vi "Init.vi"(5 "PathControl.lvclass":refnum<class "PathControl.lvclass">, 6 "Environmental classes":refnum<class "Instrument.lvclass">[](array[class]), 7 "XML Handler.lvclass":refnum<class "XML Handler.lvclass">, 8 "error in (no error)":errorcluster, 9 "Instruments to Use":T2(array[cluster]), 10 "Device.lvclass":refnum<class "Device.lvclass">, 11 "Measurements in":refnum<class "Measurement.lvclass">) -> (0 "error out":errorcluster, 3 "Measurements out":refnum<class "Measurement.lvclass">)   [LabVIEW 2020, in "Measurement.lvclass"]
doc: "Initializes the measurement.\nThis verifies that the instruments are present and adds them into the class data.\nIs also adds the xml handler into the class data."
uses:
  Measurement.lvclass
  Devices/Device.lvclass
  Instruments/Instrument.lvclass
  XML Handler/XML Handler.lvclass
  Path Control/PathControl.lvclass
  Path Control/Measurements Specific Paths.ctl
  Controls/Init States.ctl
  Instruments/Power Supply/Power Supply.lvclass
  Instruments/Temperature Control/Temperature Control.lvclass
  Instruments/Digital Multimeter/Digital Multimeter.lvclass
  Measurement.lvclass/Measurement.ctl
  Devices/Controls/Change setting mode enum.ctl
  Devices/PIC-device/PIC-Device.lvclass
panel:
  in  "Measurement specific paths":T1=enum."IMD"
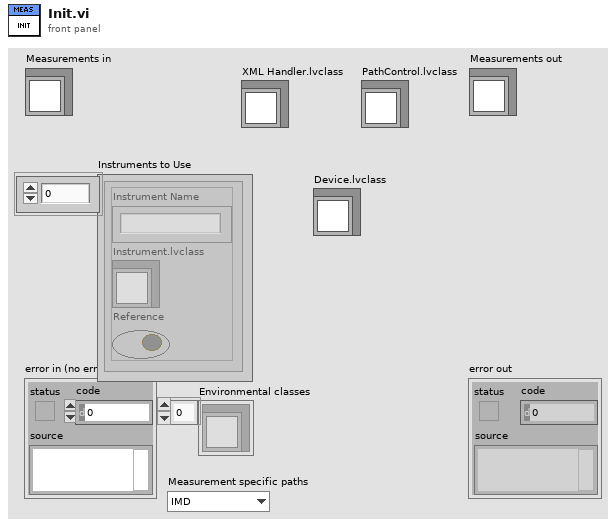
[diagram p1: front panel]
types:
  T1 = typedef "PathControl.lvclass/Measurements Specific Paths.ctl" = enum16{"No calibration", "Harmonics", "IMD", "S Parameter", "AM-AM", "MCCW-ACLR", "DC", "LCR", "Power Meter GUI", "RF Power"}
  T2 = cluster{"Instrument Name":string, "Instrument.lvclass":refnum<class "Instrument.lvclass">, "Reference":bool}[]
  T3 = typedef "Measurement.lvclass/Init States.ctl" = enum16{"Verify instruments", "Init Parameters", "Init Instruments", "Add Device", "Init Device", "Create test in XML", "Set path", "Done"}
  T4 = typedef "PIC-Device.lvclass/Change setting mode enum.ctl" = enum16{"Init", "Next", "Reset"}
  T5 = typedef "Device.lvclass/DC Offset Cluster.ctl" = cluster{"Enable":bool, "Use Array":bool, "Array":dbl[], "To From Cluster":cluster{"From":dbl, "To":dbl, "Step":dbl}, "Current Value":dbl, "DC Offset":refnum<class "Power Supply.lvclass">}
  T6 = typedef "Device.lvclass/Device Information Cluster.ctl" = cluster{"Device Info":string[][], "Default Values":T7[], "Fetched info":string[][]}
  T7 = typedef "PIC-Device.lvclass/Register to Write.ctl" = cluster{"Register":u32, "Value":u32, "Dev Address":u32, "Physical Adress":u32}
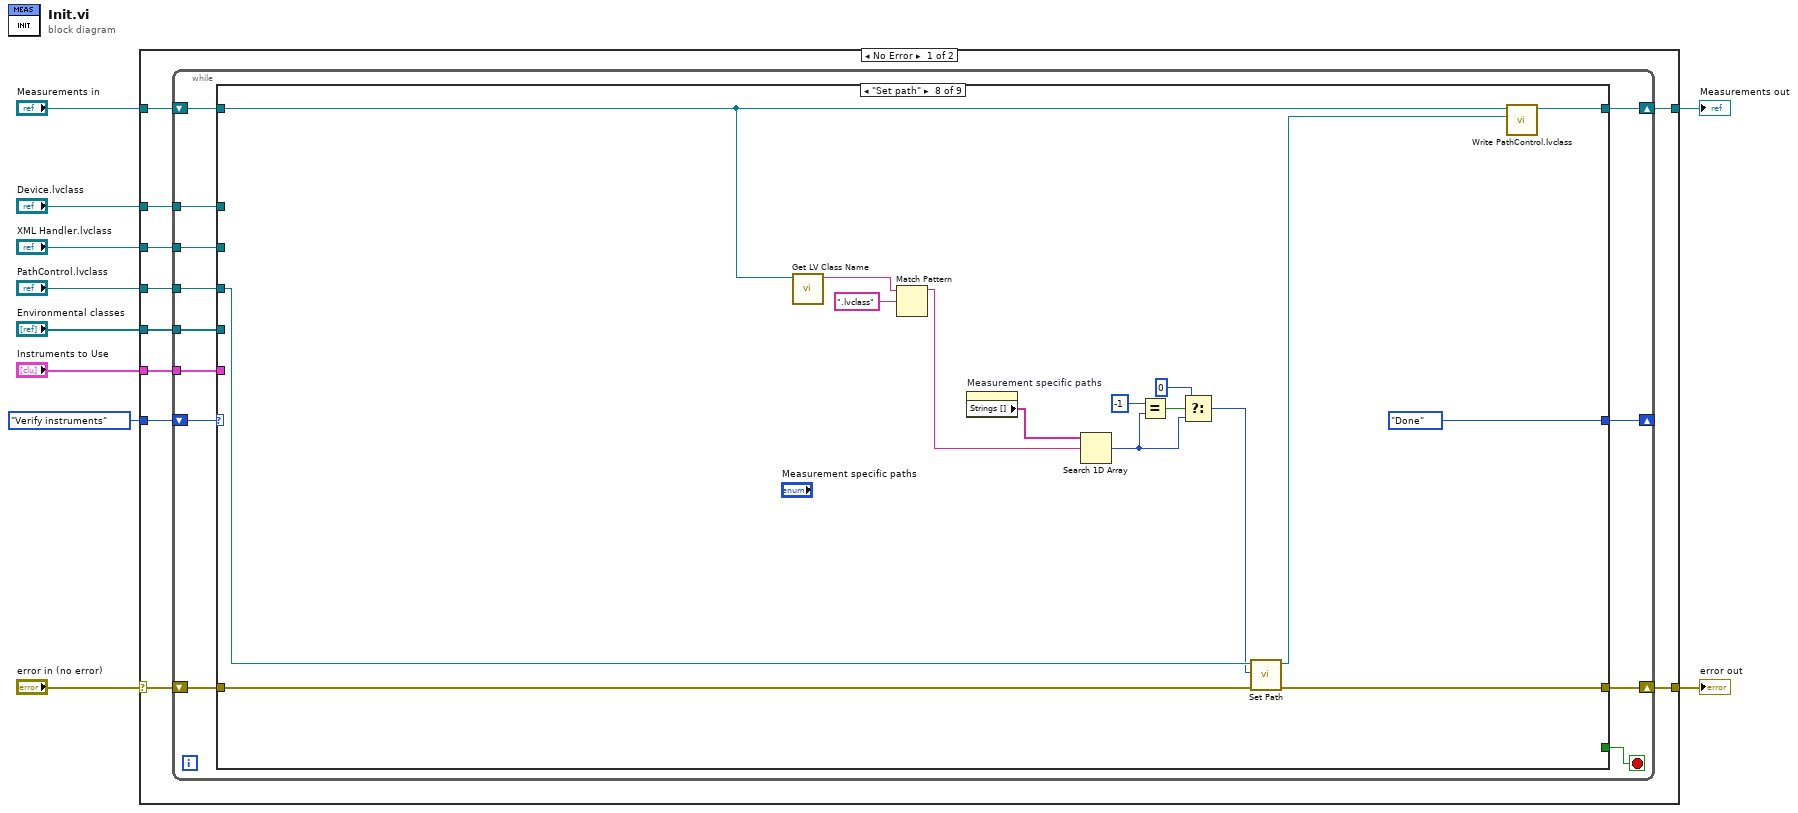
[diagram p0: block diagram]
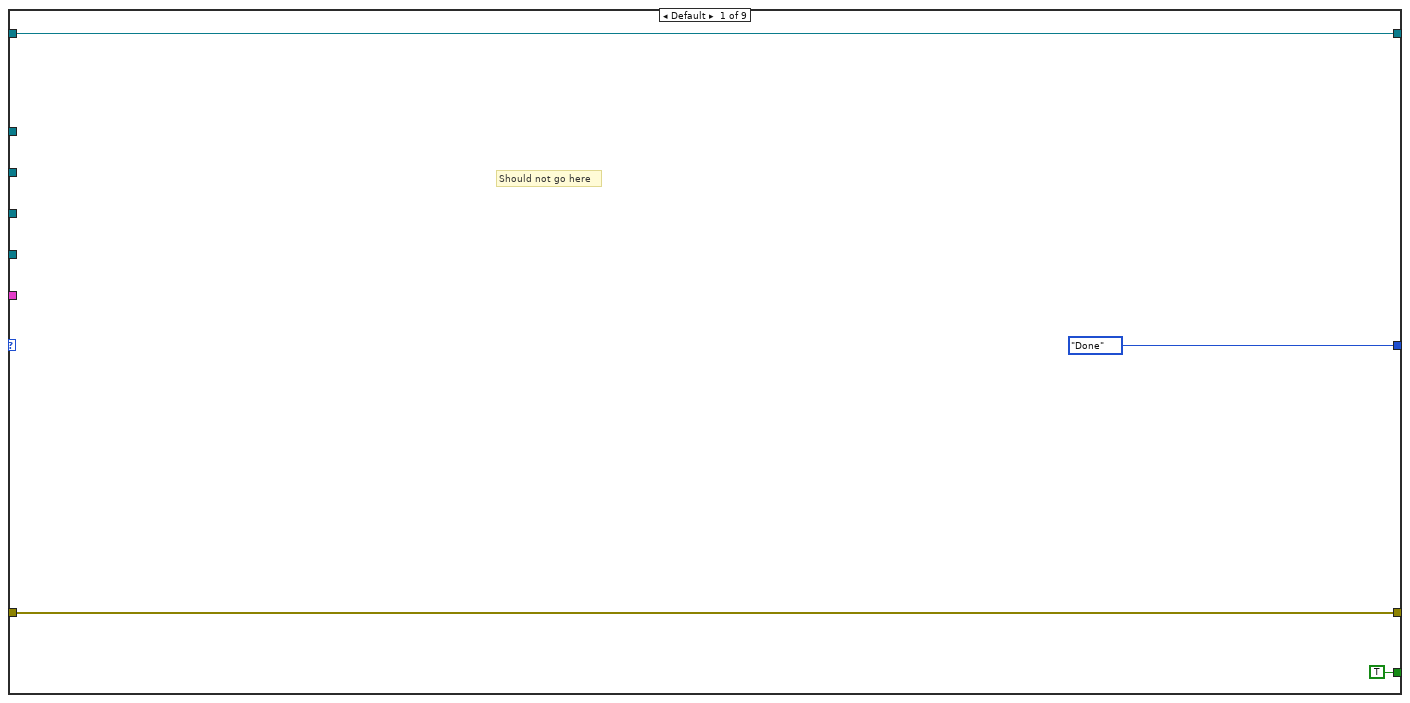
[diagram p2: hidden frame]
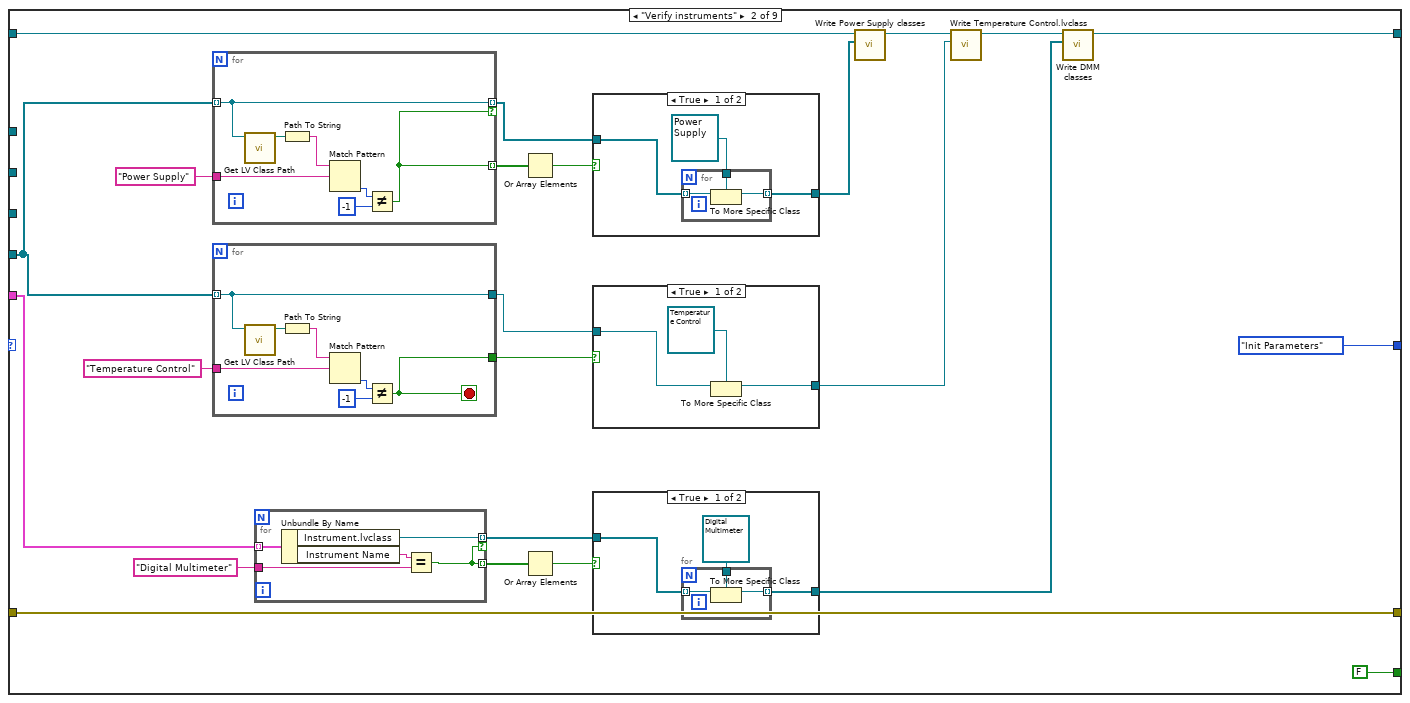
[diagram p3: hidden frame]
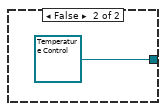
[diagram p4: hidden frame]
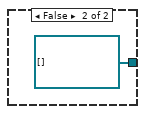
[diagram p5: hidden frame]
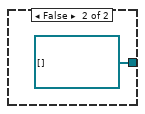
[diagram p6: hidden frame]
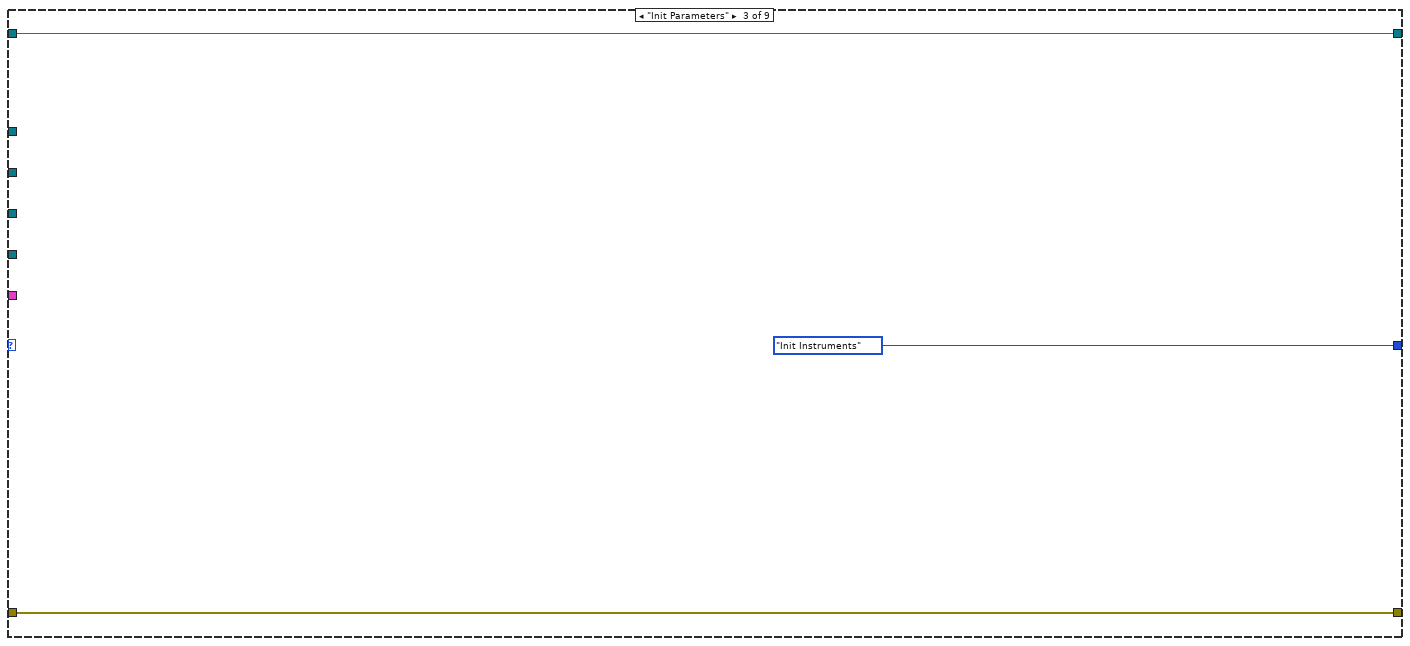
[diagram p7: hidden frame]
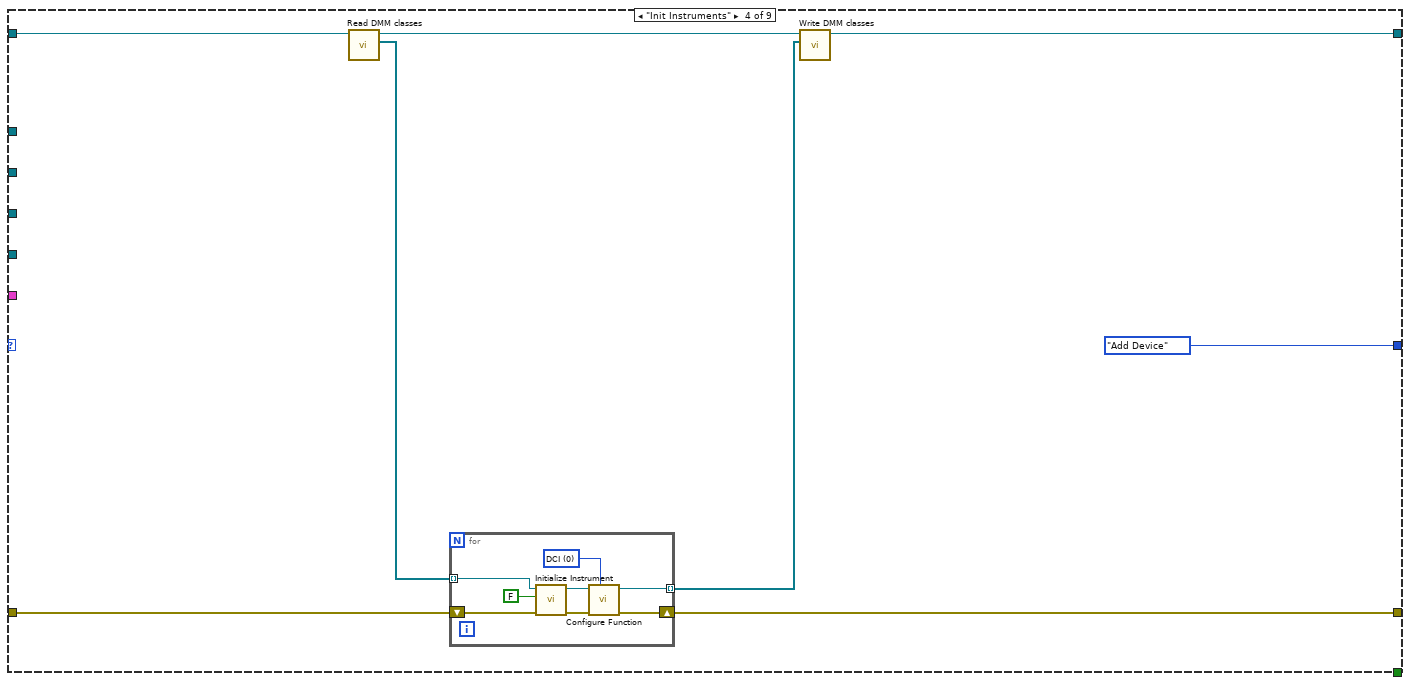
[diagram p8: hidden frame]
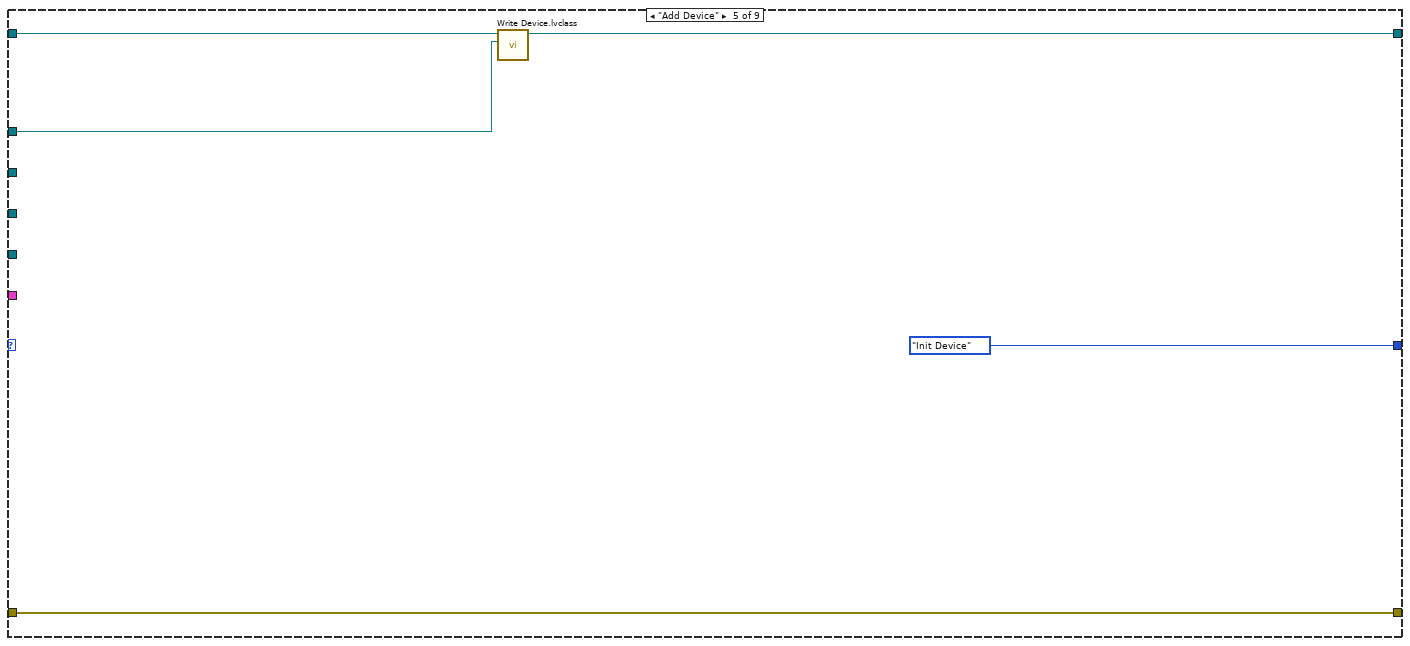
[diagram p9: hidden frame]
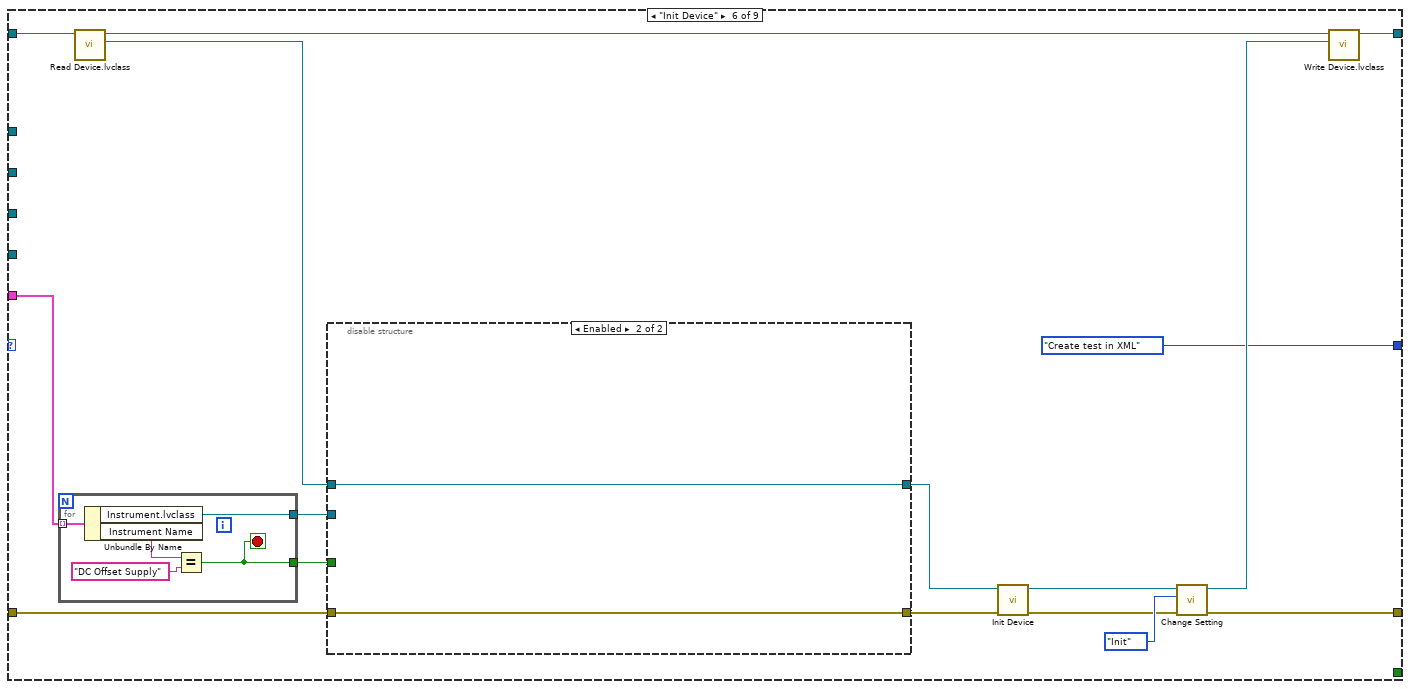
[diagram p10: hidden frame]
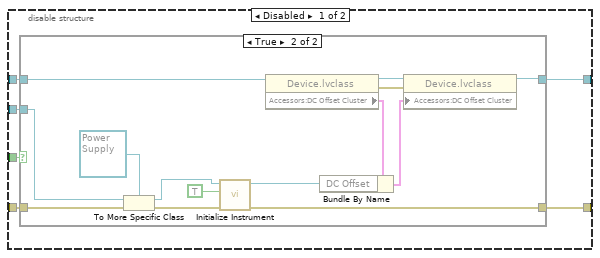
[diagram p11: hidden frame]
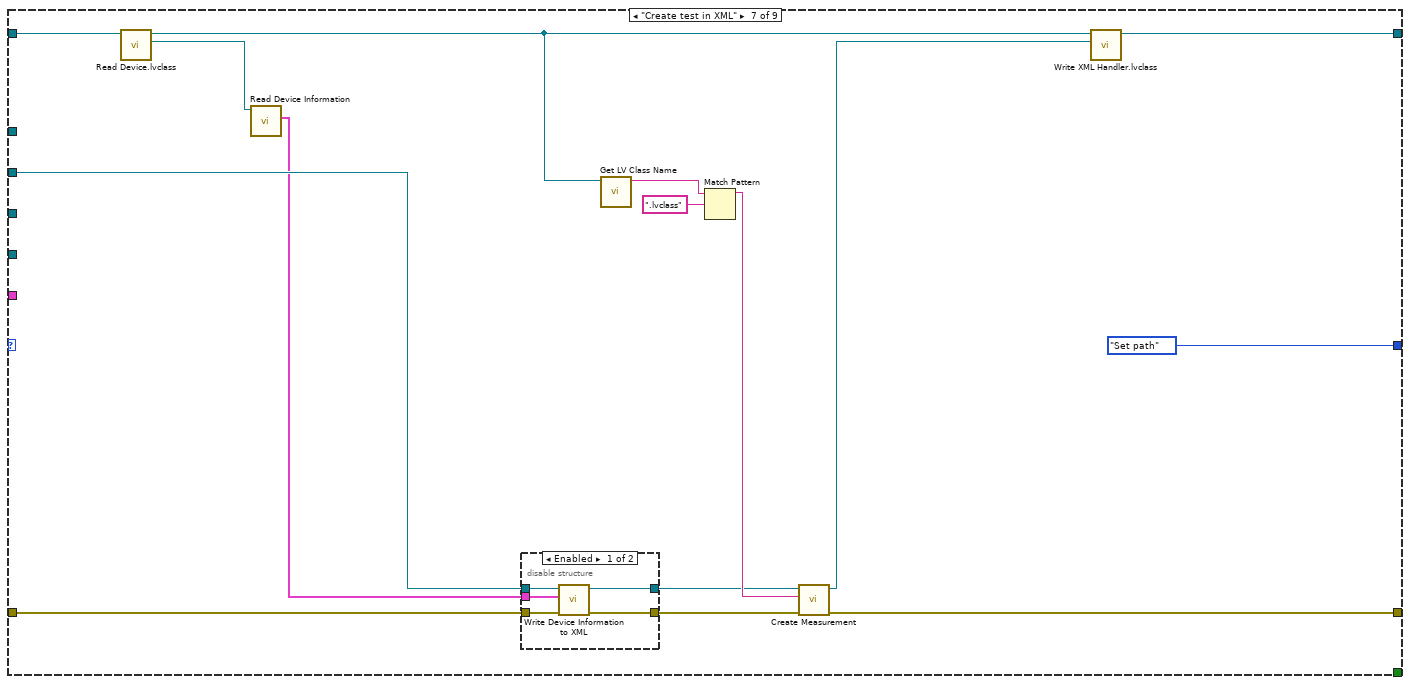
[diagram p13: hidden frame]
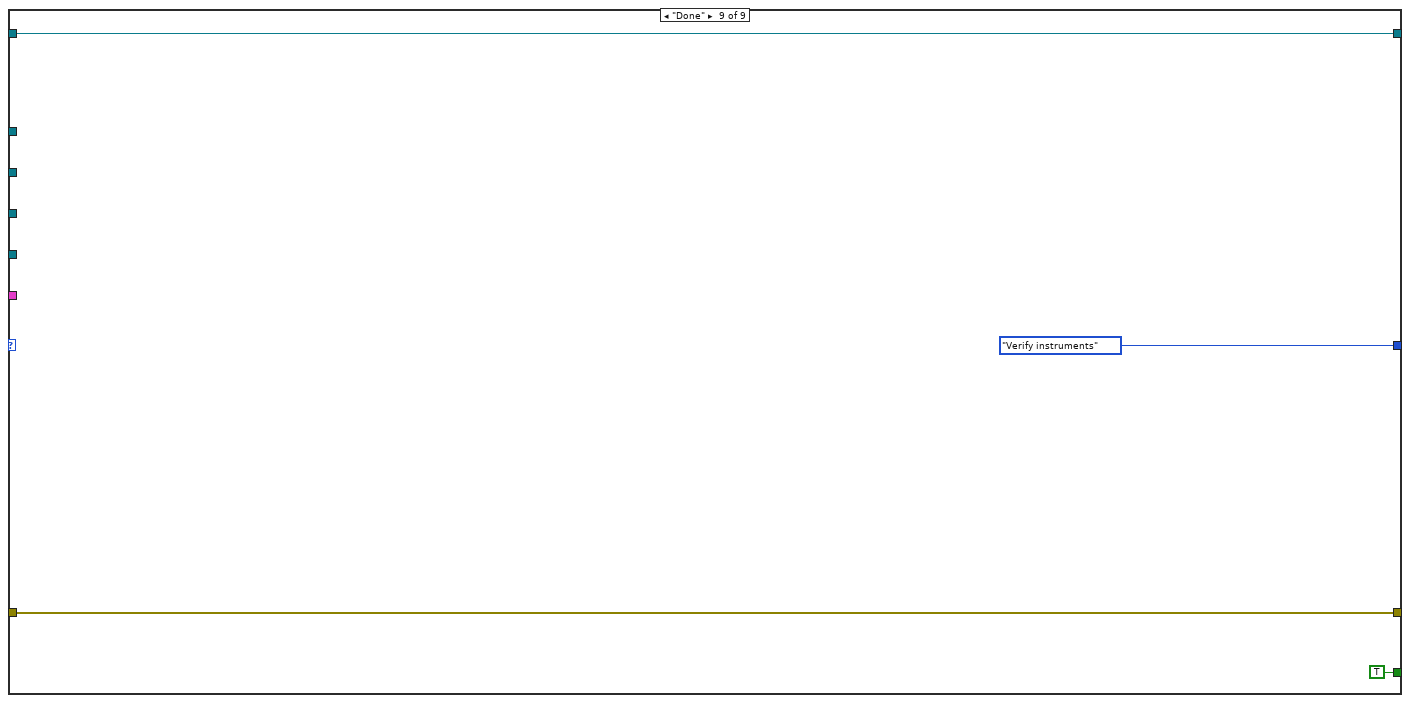
[diagram p15: hidden frame]
diagram:
  n1 = case shown="No Error" "error in (no error)" {
    selector: "error in (no error)" -> [w18 w209]
    tunnel: [w17 w209] -> w9
    tunnel: [w19 w208] -> w7
    tunnel: "Measurements in" -> [w20 w208]
    tunnel: Init_States."Verify instruments" -> [w11 _]
    tunnel: "Instruments to Use" -> [w16 _]
    tunnel: "Environmental classes" -> [w15 _]
    tunnel: "Device.lvclass" -> [w14 _]
    tunnel: "XML Handler.lvclass" -> [w13 _]
    tunnel: "PathControl.lvclass" -> [w12 _]
    frame No Error {
      n2 = while {
        shift-right: [w29] -> w19
        shift-left: w20 -> [w31]
        shift-right: [w28] -> w17
        shift-left: w18 -> [w32]
        tunnel: w16 -> [w27]
        tunnel: w15 -> [w26]
        shift-right: [w24] -> _
        shift-left: w11 -> [w30]
        tunnel: w14 -> [w23]
        tunnel: w13 -> [w22]
        tunnel: w12 -> [w21]
        stop <- w25 stop-if-true
        n3 = case shown="\"Set path\"" w30 {
          tunnel: w32 -> [w35 w47 w99 w104 w118 w125 w171 w201 w206]
          tunnel: w31 -> [w36 w55 w98 w102 w120 w127 w170 w196 w207]
          tunnel: [w36 w38 w98 w101 w119 w128 w179 w202 w207] -> w29
          tunnel: [w35 w47 w99 w103 w118 w124 w175 w200 w206] -> w28
          tunnel: w27 -> [_ w56 _ _ _ w126 _ _ _]
          tunnel: w26 -> [_ w43 _ _ _ _ _ _ _]
          tunnel: [TRUE FALSE _ _ _ _ _ _ TRUE] -> w25
          tunnel: [Init_States."Done" Init_States."Init Parameters" Init_States."Init Instruments" Init_States."Add Device" Init_States."Init Device" Init_States."Create test in XML" Init_States."Set path" Init_States."Done" Init_States."Verify instruments"] -> w24
          tunnel: w23 -> [_ _ _ _ w117 _ _ _ _]
          tunnel: w22 -> [_ _ _ _ _ _ w173 _ _]
          tunnel: w21 -> [_ _ _ _ _ _ _ w199 _]
          frame Default {
            # "Should not go here"
          }
          frame "Verify instruments" {
            n4 = for {
              tunnel: "Power Supply" -> [w74]
              tunnel: [w71] -> w48 mode=indexing
              tunnel: [w77] -> w52 mode=indexing if=w71
              tunnel: w43 -> [w77] mode=indexing
              n5 = call <vilib>:"Get LV Class Path.vi"("object"=w77) -> ("class path"=w75:path)  [unwired: 9 in, 1 out]
              n6 = Path To String(path=w75) -> (string=w76:string)
              n7 = Match Pattern(string=w76, regular expression=w74) -> (offset past match=w73:i32)  [unwired: 1 in, 3 out]
              n8 = Not Equal?(x=w73, y=-1) -> (x != y?=w71:bool)
            }
            n9 = for {
              tunnel: "Temperature Control" -> [w63]
              tunnel: [w60] -> w46
              tunnel: [w66] -> w45
              tunnel: w43 -> [w66] mode=indexing
              stop <- w60 stop-if-true
              n10 = call <vilib>:"Get LV Class Path.vi"("object"=w66) -> ("class path"=w64:path)  [unwired: 9 in, 1 out]
              n11 = Path To String(path=w64) -> (string=w65:string)
              n12 = Match Pattern(string=w65, regular expression=w63) -> (offset past match=w62:i32)  [unwired: 1 in, 3 out]
              n13 = Not Equal?(x=w62, y=-1) -> (x != y?=w60:bool)
            }
            n14 = for {
              tunnel: w56 -> [w96] mode=indexing
              tunnel: "Digital Multimeter" -> [w94]
              tunnel: [w93] -> w58 mode=indexing if=w92
              tunnel: [w92] -> w51 mode=indexing
              n15 = Unbundle By Name(w96) -> ("Instrument.lvclass"=w93:refnum<class "Instrument.lvclass">, "Instrument Name"=w95:string)
              n16 = Equal?(x=w95, y=w94) -> (x = y?=w92:bool)
            }
            n17 = Or Array Elements(Boolean array=w48) -> (logical OR=w49:bool)
            n18 = Or Array Elements(Boolean array=w51) -> (logical OR=w50:bool)
            n19 = case shown="True" w49 {
              tunnel: w52 -> [w80 _]
              tunnel: [w79 refnum<class "Power Supply.lvclass">[] []] -> w54
              frame True {
                n20 = for {
                  tunnel: refnum<class "Power Supply.lvclass"> refnum ("Power Supply.lvclass") -> [w83]
                  tunnel: w80 -> [w82] mode=indexing
                  tunnel: [w81] -> w79 mode=indexing
                  n21 = To More Specific Class(target class=w83, reference=w82) -> (specific class reference=w81:refnum<class "Power Supply.lvclass">)  [unwired: 1 in, 1 out]
                }
              }
              frame False {
              }
            }
            n22 = case shown="True" w46 {
              tunnel: w45 -> [w69 _]
              tunnel: [w68 refnum<class "Temperature Control.lvclass"> refnum ("Temperature Control.lvclass")] -> w42
              frame True {
                n23 = To More Specific Class(target class=refnum<class "Temperature Control.lvclass"> refnum ("Temperature Control.lvclass"), reference=w69) -> (specific class reference=w68:refnum<class "Temperature Control.lvclass">)  [unwired: 1 in, 1 out]
              }
              frame False {
              }
            }
            n24 = case shown="True" w50 {
              tunnel: w58 -> [w86 _]
              tunnel: [w85 refnum<class "Digital Multimeter.lvclass">[] []] -> w57
              frame True {
                n25 = for {
                  tunnel: refnum<class "Digital Multimeter.lvclass"> refnum ("Digtal Multimeter.lvclass") -> [w90]
                  tunnel: w86 -> [w89] mode=indexing
                  tunnel: [w88] -> w85 mode=indexing
                  n26 = To More Specific Class(target class=w90, reference=w89) -> (specific class reference=w88:refnum<class "Digital Multimeter.lvclass">)  [unwired: 1 in, 1 out]
                }
              }
              frame False {
              }
            }
            n27 = call-dynamic "Write Power Supply classes.vi"("Power Supply classes"=w54, "Measurements in"=w55) -> ("Measurements out"=w40:refnum<class "Measurement.lvclass">)  [unwired: 9 in]
            n28 = call-dynamic "Write Temperature Control.lvclass.vi"("Temperature Control.lvclass"=w42, "Measurements in"=w40) -> ("Measurements out"=w39:refnum<class "Measurement.lvclass">)  [unwired: 9 in]
            n29 = call-dynamic "Write DMM classes.vi"("DMM classes"=w57, "Measurements in"=w39) -> ("Measurements out"=w38:refnum<class "Measurement.lvclass">)  [unwired: 9 in]
          }
          frame "Init Parameters" {
          }
          frame "Init Instruments" {
            n30 = call-dynamic "Read DMM classes.vi"("Measurements in"=w102) -> ("DMM classes"=w107:refnum<class "Digital Multimeter.lvclass">[], "Measurements out"=w105:refnum<class "Measurement.lvclass">)  [unwired: 9 in]
            n31 = for {
              tunnel: w107 -> [w113] mode=indexing
              tunnel: [w110] -> w106 mode=indexing
              shift-right: [w109] -> w103
              shift-left: w104 -> [w115]
              w108 = u16 0 items=["DCI", "DCV"] ("Function")
              n32 = call-dynamic "Initialize Instrument.vi"("error in (no error)"=w115, "Reset"=FALSE, "Instrument in"=w113) -> ("error out"=w112:errorcluster, "Instrument out"=w111:refnum<class "Digital Multimeter.lvclass">)  [unwired: 7 in]
              n33 = call-dynamic "Configure Function.vi"("Function"=w108, "error in (no error)"=w112, "Digital Multimeter in"=w111) -> ("error out"=w109:errorcluster, "Digital Multimeter out"=w110:refnum<class "Digital Multimeter.lvclass">)  [unwired: 7 in]
            }
            n34 = call-dynamic "Write DMM classes.vi"("DMM classes"=w106, "Measurements in"=w105) -> ("Measurements out"=w101:refnum<class "Measurement.lvclass">)  [unwired: 9 in]
          }
          frame "Add Device" {
            n35 = call "Write Device.lvclass.vi"("Device.lvclass"=w117, "Measurements in"=w120) -> ("Measurements out"=w119:refnum<class "Measurement.lvclass">)  [unwired: 9 in]
          }
          frame "Init Device" {
            n36 = for {
              tunnel: w126 -> [w164] mode=indexing
              tunnel: [w162] -> w131
              tunnel: [w161] -> w130
              stop <- w162 stop-if-true
              n37 = Unbundle By Name(w164) -> ("Instrument.lvclass"=w161:refnum<class "Instrument.lvclass">, "Instrument Name"=w163:string)
              n38 = Equal?(x=w163, y="DC Offset Supply") -> (x = y?=w162:bool)
            }
            n39 = call "Read Device.lvclass.vi"("Measurements in"=w127) -> ("Device.lvclass"=w133:refnum<class "Device.lvclass">, "Measurements out"=w135:refnum<class "Measurement.lvclass">)  [unwired: 9 in]
            n40 = disable-structure shown="Enabled" {
              disable-tunnel: w133 -> [w142 w160]
              disable-tunnel: [w141 w160] -> w132
              disable-tunnel: w131 -> [w140 _]
              disable-tunnel: w130 -> [w139 _]
              disable-tunnel: [w138 w159] -> w129
              disable-tunnel: w125 -> [w137 w159]
              frame Disabled {
                n41 = case shown="True" w140 {
                  tunnel: w142 -> [w144 w148]
                  tunnel: [w144 w147] -> w141
                  tunnel: w139 -> [_ w158]
                  tunnel: w137 -> [w143 w151]
                  tunnel: [w143 w153] -> w138
                  frame False {
                  }
                  frame True {
                    n42 = To More Specific Class(target class=refnum<class "Power Supply.lvclass"> refnum ("Power Supply.lvclass"), reference=w158, error in=w151) -> (specific class reference=w156:refnum<class "Power Supply.lvclass">, error out=w152:errorcluster)
                    n43 = call-dynamic "Initialize Instrument.vi"("error in (no error)"=w152, "Reset"=TRUE, "Power Supply in"=w156) -> ("error out"=w153:errorcluster, "Power Supply out"=w155:refnum<class "Power Supply.lvclass">)  [unwired: 7 in]
                    n44 = property class="Device.lvclass"(reference=w148) -> (reference out=w149:refnum<class "Device.lvclass">, error out=w150:errorcluster, "Accessors:DC Offset Cluster"=w145:T5)  [unwired: 1 in]
                    n45 = Bundle By Name(cluster=w145, "DC Offset"=w155) -> (w146:T5)
                    n46 = property class="Device.lvclass"(reference=w149, error in=w150, "Accessors:DC Offset Cluster"=w146) -> (reference out=w147:refnum<class "Device.lvclass">)  [unwired: 1 out]
                  }
                }
              }
              frame Enabled {
              }
            }
            n47 = call-dynamic "Init Device.vi"("error in (no error)"=w129, "Device in"=w132) -> ("error out"=w123:errorcluster, "Device out"=w122:refnum<class "Device.lvclass">)  [unwired: 8 in]
            n48 = call-dynamic "Change Setting.vi"("error in (no error)"=w123, "Change setting mode"=Change_setting_mode_enum."Init", "Device in"=w122) -> ("error out"=w124:errorcluster, "Device out"=w134:refnum<class "Device.lvclass">)  [unwired: 5 in, 2 out]
            n49 = call "Write Device.lvclass.vi"("Device.lvclass"=w134, "Measurements in"=w135) -> ("Measurements out"=w128:refnum<class "Measurement.lvclass">)  [unwired: 9 in]
          }
          frame "Create test in XML" {
            n50 = call "Read Device.lvclass.vi"("Measurements in"=w170) -> ("Device.lvclass"=w168:refnum<class "Device.lvclass">, "Measurements out"=w169:refnum<class "Measurement.lvclass">)  [unwired: 9 in]
            n51 = call-dynamic "Read Device Information.vi"("Device in"=w168) -> ("Device Info"=w167:T6[])  [unwired: 8 in, 2 out]
            n52 = disable-structure shown="Enabled" {
              disable-tunnel: [w185 w186] -> w174
              disable-tunnel: w173 -> [w184 w186]
              disable-tunnel: [w183 w187] -> w172
              disable-tunnel: w171 -> [w182 w187]
              disable-tunnel: w167 -> [w181 _]
              frame Enabled {
                n53 = call "Write Device Information to XML.vi"("error in (no error)"=w182, "Device Information"=w181, "XML Handler in"=w184) -> ("error out"=w183:errorcluster, "XML Handler out"=w185:refnum<class "XML Handler.lvclass">)  [unwired: 7 in]
              }
              frame Disabled {
              }
            }
            n54 = call <vilib>:"Get LV Class Name.vi"("object"=w169) -> ("class name"=w177:string)  [unwired: 9 in, 1 out]
            n55 = Match Pattern(string=w177, regular expression=".lvclass" ("string")) -> (before substring=w176:string)  [unwired: 1 in, 3 out]
            n56 = call "Create Measurement.vi"("error in (no error)"=w172, "Measurement Name"=w176, "XML Handler in"=w174) -> ("error out"=w175:errorcluster, "XML Handler out"=w180:refnum<class "XML Handler.lvclass">)  [unwired: 7 in]
            n57 = call "Write XML Handler.lvclass.vi"("XML Handler.lvclass"=w180, "Measurements in"=w169) -> ("Measurements out"=w179:refnum<class "Measurement.lvclass">)  [unwired: 9 in]
          }
          frame "Set path" {
            n58 = call <vilib>:"Get LV Class Name.vi"("object"=w196) -> ("class name"=w197:string)  [unwired: 9 in, 1 out]
            n59 = Match Pattern(string=w197, regular expression=".lvclass" ("string")) -> (before substring=w195:string)  [unwired: 1 in, 3 out]
            n60 = property on="Measurement specific paths" class="Enum (strict)"() -> ("Strings []"=w194:string[])  [unwired: 2 in, 2 out]
            n61 = Search 1D Array(1D array=w194, element=w195) -> (index of element=w191:i32)  [unwired: 1 in]
            n62 = Equal?(x=-1 ("y"), y=w191) -> (x = y?=w192:bool)
            n63 = Select(t=0, s=w192, f=w191) -> (s? t:f=w190:i32)
            n64 = call "Set Path.vi"("error in (no error)"=w201, "Measurement specfic paths"=w190, "PathControl in"=w199) -> ("error out"=w200:errorcluster, "PathControl out"=w203:refnum<class "PathControl.lvclass">)  [unwired: 7 in]
            n65 = call "Write PathControl.lvclass.vi"("PathControl.lvclass"=w203, "Measurements in"=w196) -> ("Measurements out"=w202:refnum<class "Measurement.lvclass">)  [unwired: 9 in]
          }
          frame "Done" {
          }
        }
      }
    }
    frame Error {
    }
  }
  "error out" <- w9
  "Measurements out" <- w7
